vi "Blend U8.vi"(5 "Back":u32(colorbox)=16448250, 6 "Alpha":u8=255, 7 "Front":u32(colorbox), 11 "U8":u8[][](array[numeric])) -> (3 "image data":T1)   [LabVIEW 2023, in "Glyph Drawer.lvlib"]
uses:
  Glyph/Glyph Drawer.lvlib
  <vilib>/picture/picture.llb/imagedata.ctl
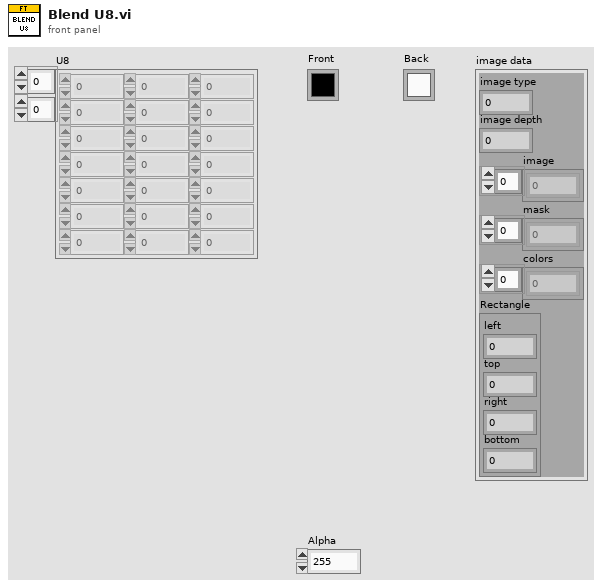
[diagram p1: front panel]
types:
  T1 = typedef "imagedata.ctl" = cluster{"image type":i32, "image depth":i32, "image":u8[], "mask":u8[], "colors":u32[], "Rectangle":cluster{"left":i16, "top":i16, "right":i16, "bottom":i16}}
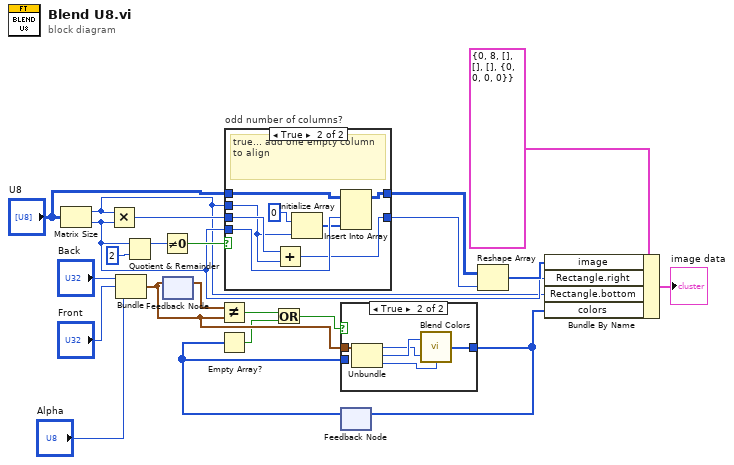
[diagram p0: block diagram]
diagram:
  n1 = Matrix Size(0:"U8") -> (1:w11:i32, 2:w12:i32)
  n2 = Multiply(x=w11, y=w12) -> (x*y=w20:i32)
  n3 = Bundle("Back"="Back", "Front"="Front", "Alpha"="Alpha") -> (w8:cluster{"Back":u32, "Front":u32, "Alpha":u8})  [unwired: 1 in]
  n4 = Quotient & Remainder(x=w12, y=2) -> (x-y*floor(x/y)=w17:i32)  [unwired: 1 out]
  n5 = Not Equal To 0?(x=w17) -> (x != 0?=w14:bool)
  n6 = feedback-in #1(w8) -> ()
  n7 = feedback #1() -> (w7:cluster{"Back":u32, "Front":u32, "Alpha":u8})  [unwired: 1 in]
  n8 = Not Equal?(x=w7, y=w8) -> (x != y?=w5:bool)
  n9 = case "odd number of columns?" shown="True" w14 {
    tunnel: w20 -> [w23 w32]
    tunnel: "U8" -> [w24 w31]
    tunnel: [w24 w30] -> w16
    tunnel: w12 -> [_ w29]
    tunnel: [w23 w26] -> w15
    tunnel: w11 -> [_ w25]
    frame False {
    }
    frame True {
      # "true... add one empty column to align"
      n10 = Add(x=w32, y=w25) -> (x+y=w26:i32)
      n11 = Initialize Array(u8 0, w25) -> (w27:u8[])
      n12 = Insert Into Array(array=w31, index (col)=w29, new element=w27) -> (w30:u8[][])  [unwired: 1 in]
    }
  }
  n13 = feedback #2() -> (w3:u32[])  [unwired: 1 in]
  n14 = Empty Array?(array=w3) -> (empty?=w2:bool)
  n15 = Or(x=w5, y=w2) -> (x .or. y?=w4:bool)
  n16 = case shown="True" w4 {
    tunnel: w8 -> [_ w38]
    tunnel: [w33 w37] -> w6
    tunnel: w3 -> [w33 _]
    frame False {
    }
    frame True {
      n17 = Unbundle(w38) -> ("Back"=w35:u32, "Front"=w36:u32, "Alpha"=w34:u8)
      n18 = call "Blend Colors.vi"("Alpha"=w34, "Target"=w35, "Source"=w36) -> ("Array"=w37:u32[])
    }
  }
  n19 = feedback-in #2(w6) -> ()
  n20 = Reshape Array(w16, w15) -> (w19:u8[])
  n21 = Bundle By Name(cluster=T1 {"image type"=0, "image depth"=8, "image"=[], "mask"=[], "colors"=[], "Rectangle"={"left"=0, "top"=0, "right"=0, "bottom"=0}} ("image data"), "image"=w19, "Rectangle.right"=w12, "Rectangle.bottom"=w11, "colors"=w6) -> (→"image data":T1)
